vi "rqp_Start Exiting.vi"(7 "Caller in":refnum<class "Worker.lvclass">, 8 "error in":errorcluster, 11 "Fluke DMM in":refnum<class "Keithley DMM.lvclass">) -> (0 "error out":errorcluster, 3 "dup Fluke DMM out":refnum<class "Keithley DMM.lvclass">)   [LabVIEW 2020, in "Keithley DMM.lvclass"]
doc: "This VI will indirectly send a message to the <Start Exiting> MHL case of the Worker that own this VI.\n---\nThe shutdown sequence of the Worker that owns this VI will be initiated."
uses:
  Keithley DMM.lvclass
  C:/Program Files (x86)/National Instruments/LabVIEW 2020/vi.lib/addons/_Workers/Library/Classes/Worker/Worker.lvclass
  <vilib>/addons/_Workers/Library/Classes/Worker/Worker.lvclass
  <vilib>/addons/_Workers/Library/Classes/Message Queue/Message Queue.lvclass
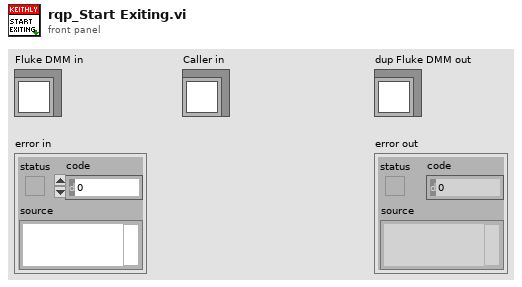
[diagram p1: front panel]
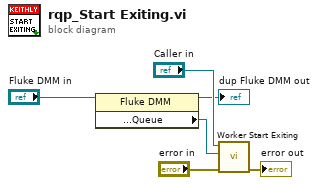
[diagram p0: block diagram]
diagram:
  n1 = property class="Fluke DMM"(reference="Fluke DMM in") -> (reference out=→"dup Fluke DMM out":refnum<class "Keithley DMM.lvclass">, "Accessors:Read:Public API:Queue"=w6:refnum<class "Message Queue.lvclass">)  [unwired: 1 in, 1 out]
  n2 = call-dynamic "Worker Start Exiting.vi"("error_in"="error in", "Message Queue"=w6, "Worker"="Caller in") -> ("error out"=→"error out":errorcluster)  [unwired: 7 in, 1 out]
